vi "WriteCustomCall.vi"(2 "Filename":string, 3 "NXT":T1={"Hardware"="NXT", "Flattened String"=""}, 8 "Custom Data":string) -> (0 "NXT":T1={"Hardware"="NXT", "Flattened String"=""})   [LabVIEW 2010, in "Packet Recorder.lvlib"]
uses:
  Packet Recorder.lvlib
  <vilib>/NXT/Subs/LVHSConnector.ctl
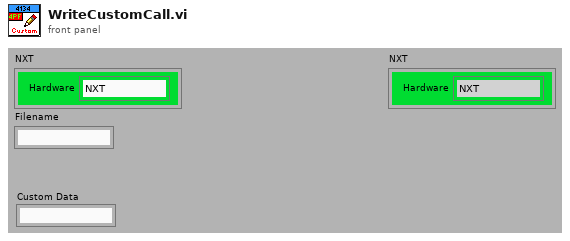
[diagram p1: front panel]
types:
  T1 = typedef "LVHSConnector.ctl" = cluster{"Hardware":string, "Flattened String":string}
  T2 = enum16{"big-endian, network order", "native, host order", "little-endian"}
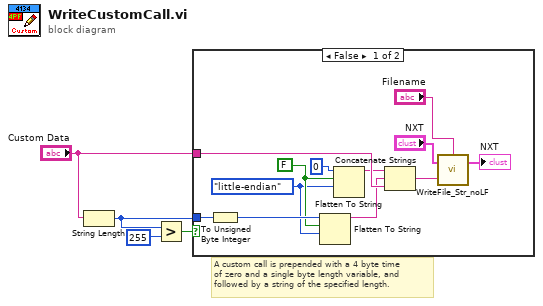
[diagram p0: block diagram]
diagram:
  # "A custom call is prepended with a 4 byte time\nof zero and a single byte length variable, and\nfollowed by a string of the specified length."
  n1 = String Length(string="Custom Data") -> (length=w1:i32)
  n2 = Greater?(x=w1, y=255) -> (0:w3:bool)
  n3 = case shown="False" w3 {
    tunnel: "Custom Data" -> [w10 _]
    tunnel: w1 -> [w12 _]
    frame False {
      w7 = FALSE ("prepend array or string size? (T)")
      w6 = T2."little-endian" ("byte order (0:big-endian, network order)")
      n4 = To Unsigned Byte Integer(number=w12) -> (unsigned 8bit integer=w11:u8)
      n5 = Flatten To String(anything=w11, prepend array or string size? (T)=w7, byte order (0:big-endian, network order)=w6) -> (data string=w9:string)  [unwired: 1 in, 2 out]
      n6 = Flatten To String(anything=0 ("length"), prepend array or string size? (T)=w7, byte order (0:big-endian, network order)=w6) -> (data string=w5:string)  [unwired: 1 in, 2 out]
      n7 = Concatenate Strings(w5, w9, w10) -> (w13:string)
      n8 = call <vilib>:"WriteFile_Str_noLF.vi"("String"=w13, "NXT"="NXT", "Filename"="Filename") -> ("NXT"=→"NXT":T1)  [unwired: 1 in]
    }
    frame True {
      # "Too long"
    }
  }
